vi "VISnipDiagram.vi"(8 "error in (no error)":errorcluster, 10 "Parameters":string[](array[string])) -> (0 "error out":errorcluster)   [LabVIEW 2013]
uses:
  VIVendor/PngSnippet/VVPngSnippet.lvlib
  VIDiagram/VIDiagram.lvlib
panel:
  # "Path to VI"
  # "Path to PNG"
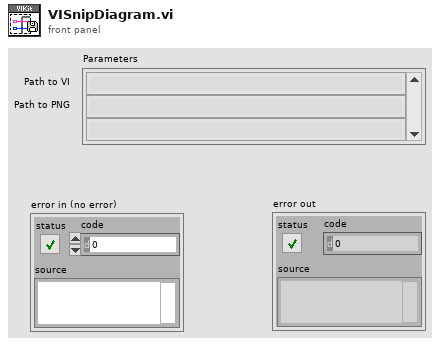
[diagram p1: front panel]
types:
  T1 = typedef "imagedata.ctl" = cluster{"image type":i32, "image depth":i32, "image":u8[], "mask":u8[], "colors":u32[], "Rectangle":cluster{"left":i16, "top":i16, "right":i16, "bottom":i16}}
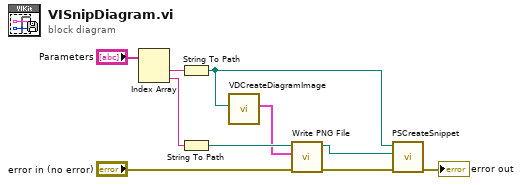
[diagram p0: block diagram]
diagram:
  n1 = Index Array(array="Parameters") -> (element #1=w5:string, element #2=w4:string)  [unwired: 2 in]
  n2 = String To Path(string=w5) -> (path=w2:path)
  n3 = String To Path(string=w4) -> (path=w8:path)
  n4 = call "VDCreateDiagramImage.vi"("VI path"=w2) -> ("image data"=w1:T1)  [unwired: 10 in]
  n5 = call <vilib>:"Write PNG File.vi"("error in (no error)"="error in (no error)", "image data"=w1, "path to PNG file"=w8) -> ("error out"=w10:errorcluster, "path"=w9:path)  [unwired: 7 in]
  n6 = call "PSCreateSnippet.vi"("error in (no error)"=w10, "PNG Path"=w9, "VI Path"=w2) -> ("error out"=→"error out":errorcluster)  [unwired: 6 in, 2 out]
